vi "AlliGator Get-Set Phasor Color Map Vertices.vi"(8 "Set/Get(F)":bool, 9 "Decay Range Exponent in":dbl, 10 "Color Array in":u32[](array[colorbox]), 11 "Vertices in":cluster{"X":dbl, "Y":dbl}[](array[cluster])) -> (0 "Empty?":bool, 1 "Decay Range Exponent out":dbl, 2 "Color Array out":u32[](array[colorbox]), 3 "Vertices out":cluster{"X":dbl, "Y":dbl}[](array[cluster]))   [LabVIEW 2021, in "AlliGator Phasor Plot Color Map.lvlib"]
doc: "Stores color map vertices and their colors."
uses:
  AlliGator Phasor Plot Color Map.lvlib
panel:
  # "see the AlliGator License on the block diagram (Ctrl+E or Window:Show Block Diagram)"
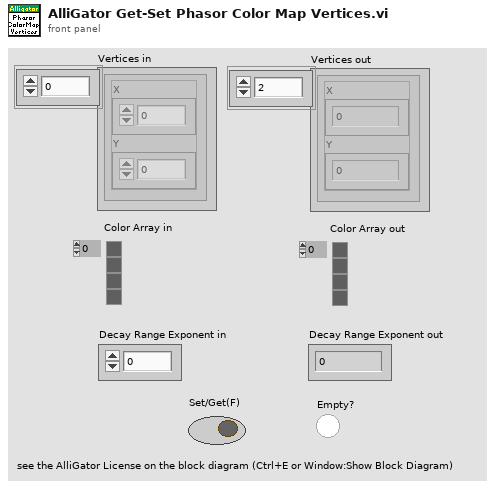
[diagram p1: front panel]
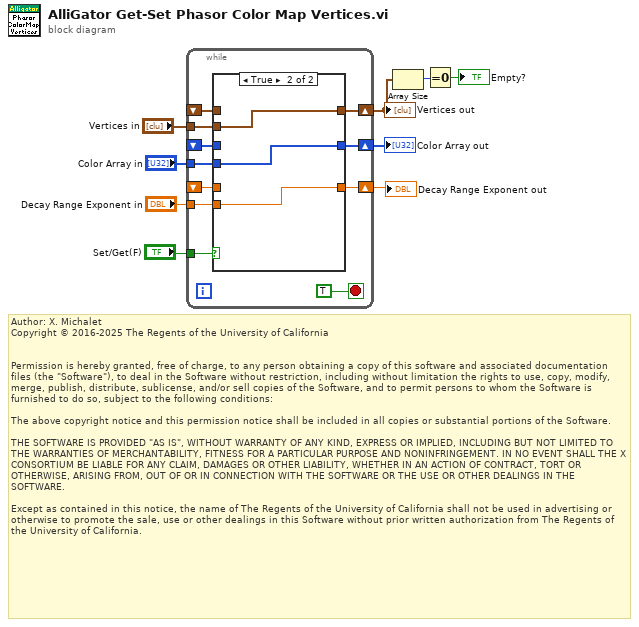
[diagram p0: block diagram]
diagram:
  # "Author: X. Michalet\nCopyright © 2016-2025 The Regents of the University of California\n \n\nPermission is hereby granted, free of charge, to any person obtaining a copy of this software and associated documentation files (the \"Software\"), to deal in the Software without restriction, including without limitation the rights to use, copy, modify, merge, publish, distribute, sublicense, and/or sell copies of the Software, and to permit persons to whom the Software is furnished to do so, subject to the following conditions:\n\nThe above copyright notice and this permission notice shall be included in all copies or substantial portions of the Software.\n\nTHE SOFTWARE IS PROVIDED \"AS IS\", WITHOUT WARRANTY OF ANY KIND, EXPRESS OR IMPLIED, INCLUDING BUT NOT LIMITED TO THE WARRANTIES OF MERCHANTABILITY, FITNESS FOR A PARTICULAR PURPOSE AND NONINFRINGEMENT. IN NO EVENT SHALL THE X CONSORTIUM BE LIABLE FOR ANY CLAIM, DAMAGES OR OTHER LIABILITY, WHETHER IN AN ACTION OF CONTRACT, TORT OR OTHERWISE, ARISING FROM, OUT OF OR IN CONNECTION WITH THE SOFTWARE OR THE USE OR OTHER DEALINGS IN THE SOFTWARE.\n\nExcept as contained in this notice, the name of The Regents of the University of California shall not be used in advertising or otherwise to promote the sale, use or other dealings in this Software without prior written authorization from The Regents of the University of California."
  n1 = while {
    tunnel: "Set/Get(F)" -> [w20]
    shift-right: [w18] -> w3
    shift-left: _ -> [w16]
    tunnel: "Vertices in" -> [w19]
    shift-right: [w15] -> w6
    shift-left: _ -> [w13]
    tunnel: "Color Array in" -> [w14]
    shift-right: [w12] -> w5
    shift-left: _ -> [w10]
    tunnel: "Decay Range Exponent in" -> [w11]
    stop <- TRUE stop-if-true
    n2 = case shown="True" w20 {
      tunnel: w19 -> [_ w26]
      tunnel: [w23 w26] -> w18
      tunnel: w16 -> [w23 _]
      tunnel: [w22 w25] -> w15
      tunnel: w14 -> [_ w25]
      tunnel: w13 -> [w22 _]
      tunnel: [w21 w24] -> w12
      tunnel: w11 -> [_ w24]
      tunnel: w10 -> [w21 _]
      frame False {
      }
      frame True {
      }
    }
  }
  "Vertices out" <- w3
  "Color Array out" <- w6
  "Decay Range Exponent out" <- w5
  n3 = Array Size(array=w3) -> (size(s)=w2:i32)
  n4 = Equal To 0?(x=w2) -> (x = 0?=→"Empty?":bool)
